vi "OrderBook-Test-1.vi"() -> ()   [LabVIEW 2016]
panel:
  in  "OrderRefNum":u64=12379813738319119365 format="%.0x"
  in  "Side":enum16{"Buy", "Sell"}(ring)=enum."Sell"
  in  "Command":enum16{"GetAll", "AddOrder", "DeleteOrder"}(ring)=enum."AddOrder"
  in  "# of Shares":u32=500
  in  "Price":dbl=139.52
  in  "Ticker":string="AAPL"
  out "Results":u64[](array[numeric]) format="%.0x"
  in  "error in":errorcluster
  out "Command":u64[](array[numeric]) format="%.0x"
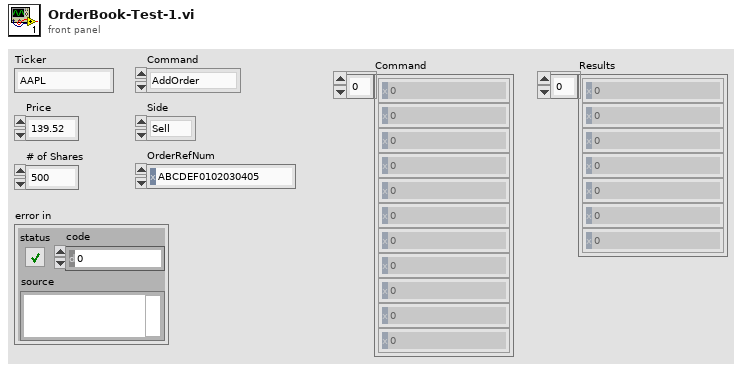
[diagram p1: front panel]
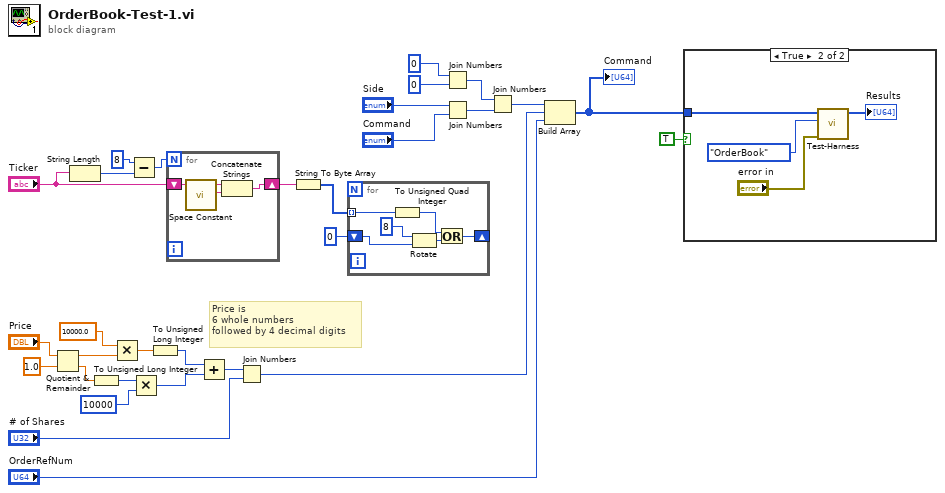
[diagram p0: block diagram]
diagram:
  # "Price is\n6 whole numbers\nfollowed by 4 decimal digits"
  n1 = Quotient & Remainder(x="Price", y=1.0) -> (x-y*floor(x/y)=w12:dbl, floor(x/y)=w11:dbl)
  n2 = String Length(string="Ticker") -> (length=w30:i32)
  n3 = To Unsigned Long Integer(number=w11) -> (unsigned 32bit integer=w6:u32)
  n4 = Multiply(x=10000.0, y=w12) -> (x*y=w10:dbl)
  n5 = Subtract(x=8, y=w30) -> (x-y=w28:i32)
  n6 = Multiply(x=w6, y=u32 10000 ("x")) -> (x*y=w7:u32)
  n7 = To Unsigned Long Integer(number=w10) -> (unsigned 32bit integer=w8:u32)
  n8 = for {
    N: w28 -> [_]
    shift-right: [w31] -> w26
    shift-left: "Ticker" -> [w33]
    n9 = call <vilib>:"Space Constant.vi"() -> ("String"=w32:string)
    n10 = Concatenate Strings(w33, w32) -> (w31:string)
  }
  n11 = Add(x=w8, y=w7) -> (x+y=w4:u32)
  n12 = Join Numbers(hi=w4, lo="# of Shares") -> ((hi.lo)=w2:u64)
  n13 = String To Byte Array(string=w26) -> (unsigned byte array=w24:u8[])
  n14 = for {
    shift-right: [w37] -> _
    shift-left: u64 0 -> [w35]
    tunnel: w24 -> [w39] mode=indexing
    n15 = To Unsigned Quad Integer(1:w39) -> (0:w36:u64)
    n16 = Rotate(1:w35, 2:i16 8 ("y")) -> (0:w38:u64)
    n17 = Or(x=w36, y=w38) -> (x .or. y?=w37:u64)
  }
  n18 = Join Numbers(hi=u16 0, lo=u16 0) -> ((hi.lo)=w19:u32)
  n19 = Join Numbers(hi="Side", lo="Command") -> ((hi.lo)=w21:u32)
  n20 = Join Numbers(hi=w19, lo=w21) -> ((hi.lo)=w20:u64)
  n21 = Build Array(w20, w2, "OrderRefNum") -> (w23:u64[])
  "Command" <- w23
  n22 = case shown="True" TRUE {
    tunnel: w23 -> [_ w41]
    frame False {
    }
    frame True {
      n23 = call "Test-Harness.vi"("error in"="error in", "Operating\nMode"=enum16{"OrderBook"}."OrderBook" ("Operating\nMode"), "DataIn"=w41) -> ("DataOut"=→"Results":u64[])  [unwired: 7 in, 1 out]
    }
  }
